vi "Forebrain.vi"() -> ()   [LabVIEW 2012]
doc: "This VI contrains the Forebrain within the Olin Robot Architecture. It must be run first to load the appropriate mission definition files. It contains a finite state machine built around a tabbed Operator interface that will guide an operator through the startup, run shutdown mission sequence. After running it, run the Midbrain and Hindbrain VIS."
panel:
  in  "Soft E-Stop":bool
  out "NXT String Received":string
  out "return count":u32
  out "error out":errorcluster
  in  "error in 2":errorcluster
  out "Desired \nVelocity":i16=5
  out "Local\nHeading":i16=90
  out "Ycurrent":dbl format="%#_3g"
  out "Xcurrent":dbl format="%#_3g"
  out "Ystart":dbl
  out "Xstart":dbl
  in  "error in":errorcluster
  out "Robot Live":bool
  in  "E-Stop":bool
  in  "Tab":T1(tab)
  out "MissionTime (Min)":dbl(knob) scale=0.0..10.0
  out "LidarDist":i16
  out "IR Index":i32
  out "BatteryLevel":dbl(slide) scale=6.0..9.0
  out "String Received":string
  out "Send String":string="$B^"
  in  "VISA resource name":refnum<visa-resource-name>="COM10"
  in  "Mode":i16 min=0 max=99 step=1
  in  "Desired Vel":i16(slide)=7 scale=0.0..14.0
  in  "Local Head":i16(slide)=7 scale=0.0..14.0
  out "StartMissionMap":picture
  out "MapDARCheck":picture
  in  "RunRobot":bool
  in  "Tug letter":string="G"
  out "Tug X":i32
  out "Tug Y":i32
  out "Tug H":i32
  out "BS Time Out?":bool
  out "Buoy locations":cluster{"regular expression":string, i32, i32}[](array[cluster])
  out "Valid ?":bool
  out "Battery\nVolts":i16
  out "Base Station data rec'd":string
  out "udp rate":bool
  out "CollisionWarning":bool
  out "DebugMapDAR":picture
  in  "MapDAR Control":T2={"NumberOfBeams"=180, "SensorRange"=500.0, "Noise (0.1 to 1)"=0.0} {"Noise (0.1 to 1)" min=0.0 max=1.0 step=0.1; "SensorRange" min=500.0 max=1500.0 step=100.0; "NumberOfBeams" min=36 max=360 step=2}
  out "MapDAR Data (r:pixel b:degrees)":cluster{"Range":dbl, "Bearing":dbl}[](array[cluster])
  in  "Stop DebugSENSE":bool
  out "MissionMap":picture
  out "Tug position":T3
  out "initialized MDF":T4(array[cluster])
  out "Way Point Index":i32
  out "InitialWaypoint":cluster{"X":i16, "Y":i16}
  in  "Pen Color":u32(colorbox)=15671808
  in  "Select Pen Attributes":T5={"Width"=1, "Style"=enum."Solid"}
  out "Draw??":bool
  in  "WhereAmI?FromBase":T6
  out "(xr,yr)":cluster{"X":dbl, "Y":dbl}
  in  "RobotPosition":T3 {"xrobot" min=0.0 max=1177.0 step=10.0; "yrobot" min=0.0 max=850.0 step=10.0; "heading" min=0.0 max=7.0 step=0.1}
  out "MDF_Original":T4(array[cluster])
  out "WhatAroundMeMap?":cluster{"T":dbl, "Range":dbl, "Bearing":dbl}[](array[cluster])
  out "WayPointAct":dbl[](array[numeric])
  out "SteerAngle":dbl
  out "MissionDefFile":picture
  out "MDF":T4(array[cluster])
  in  "Select Your Behavior":T7(ring)
  out "No. of Waypoints":i32
  in  "Exit Planning":bool
  in  "BoatSpeed for Leg":dbl(slide)=8.0 min=-9.0 max=9.0 step=1.0 scale=0.0..14.0
  out "BuildMDF":bool
  out "WayPoint Position":cluster{"X":i32, "Y":i32}
  in  "Upper Midbrain Active":bool
  out "Send String to NXT":string="$B^"
  in  "Behavior Command":T7(ring)
  out "CollisionLight":bool
  out "Where? Manual":T6
  out "ActManual":bool
  in  "Manual Heading":i16(knob) min=0 max=14 step=1
  out "MWhat?":bool
  out "Where? 2":bool
  out "How? 2":bool
  in  "ManualModeStop":bool
  out "ManualModeMapDAR":picture
  out "ManualMissionMap":picture
  out "Battery":dbl(slide) scale=0.0..8.0
  in  "Manual Vel":dbl(slide) min=0.0 max=14.0 step=1.0 scale=0.0..14.0
  out "MissionTime":dbl(knob) scale=0.0..10.0
  out "Heading":cluster{dbl, dbl}(knob)={0.0, 34.390870865624734} scale=180.0..-179.0 scale format="%#_3g"
  out "Speed":i16(knob) scale=-6.0..6.0
  out "Current Behavior":T7(ring)
  out "Robot Position":cluster{"X":dbl, "Y":dbl} {"X" format="%#_3g"; "Y" format="%#_3g"}
  out "Ready":bool
  in  "Pause":bool
  in  "Rerun MDF":bool
  out "CollisionLight 2":bool
  out "Act":bool
  out "Neo-C":bool
  out "How?":bool
  out "What?":bool
  out "A Heading":cluster{dbl, dbl}(knob)={0.0, 34.390870865624734} scale=180.0..-180.0
  out "A Speed":dbl(knob) scale=-9.0..9.0
  out "AutoBattery":dbl(slide) scale=0.0..8.0
  out "AutoModeLIDAR":picture
  out "AutoMissionMap":picture
  in  "RunAutoMode":bool
  out "MissionTimeAuto":dbl(knob) scale=0.0..60.0
  out "Where?":bool
  # "To run\nrobot,\nclick\narrow\nabove\n\nRun Robot button must be on"
  # "Operation Directions\n\n1)Click on Startup&\nShutdown tab.\n2) Click on Run \nArrow on menubar.\nRun Forebrain,\nvis from the project\nexplorer.\n3) Select a mssion \nmap file when asked.\n4) Check robot is \nfully operational on\nStartup tab.\n5) Debug with debug\ntabs as required.\n6) Select ManualMode\ntab and test drive \nrobot.\n7) Select PlanMission\ntab and set up \nmission.\n8) Go to AutoMode\ntab and run mission."
  # "Turns off drive\nmotors"
  # "Enter Olin Test  Pool"
  # "Xbee Com Port"
  # "xBee\"Send String\" (mode, desired velocity, local heading)"
  # "(Type in Tug Letter  L T G P  (look at boat cradle)"
  # "Should be on to\nrun"
  # "BoatG,X,Y,H,BoatT,X,Y,H,BoatP,X,Y.H,BoatL,X,Y,H,BuoyA,X,Y,BuoyB,X,Y,BuoyC,X,Y,BuoyD,X,Y,Time(hours,Min,Sec)"
  # "To stop  program \nturn off here"
  # "Use this tab\nto explore\nLIDAR\ndata and \noperation"
  # "Set\nNumberOfBeams\nSensorRange\nNoise\nto\nview\nsimulated\nsensor\ndata"
  # "Turn Debug Sim \nto leave this\ntab--->"
  # "This tab will auto\nreturn to Startup \nin 2 seconds"
  # "Clean up interface and make more useful for debugging behaviors"
  # "Build out interface and make more useful for debugging act"
  # "This tab will auto\nreturn to Startup \nin 2 seconds"
  # "Directions:\n1) Select Robot Behavior for each mission leg.\n2) Select Robot Speed for leg.\n3) Click on robots current location for first waypoint.\n4) Hold down button and drag to next\nwaypoint. Click on next leg waypoint.\n5) Hold mouse button down and drag to \nnext waypoint. \n6) Click on next waypoint. Repeat for full mission.\n7) MDF will store up to 20 waypoints."
  # "Remember to\nset boat\nleg speed !"
  # "Please Adjust Scroll Barrs in Tug Off Mode to Prevent  Extra Lines Being Drawn"
  # "\"Send String\" (mode, desired velocity, local heading)"
  # "Press to stop and return to StartUp"
  # "Open MidBrain\nArbiter to see\nBrain Waves"
  # "AutoMode\nAutomatically \nReturns to \nStartUp Mode"
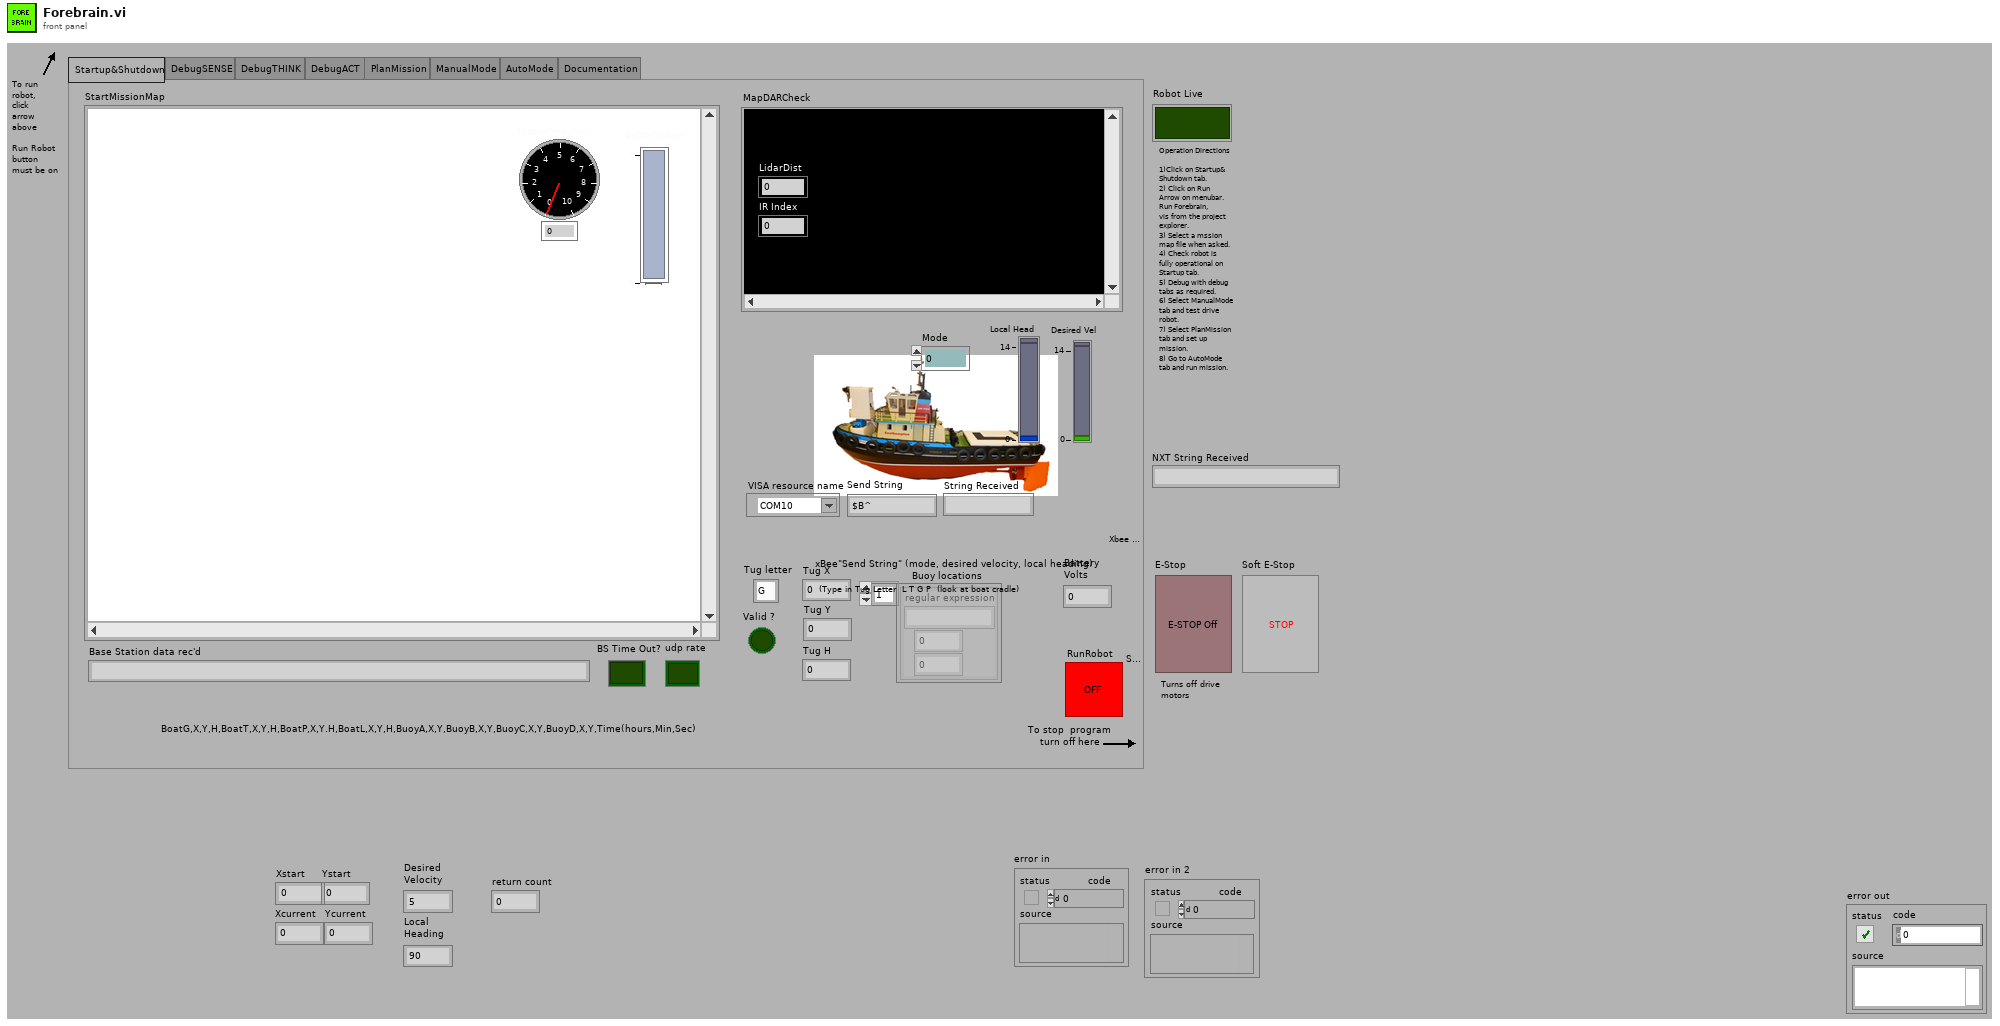
[diagram p1: front panel]
types:
  T1 = enum32{"Startup&Shutdown", "DebugSENSE", "DebugTHINK", "DebugACT", "PlanMission", "ManualMode", "AutoMode", "Documentation"}
  T2 = cluster{"NumberOfBeams":i32, "SensorRange":dbl, "Noise (0.1 to 1)":dbl}
  T3 = cluster{"xrobot":dbl, "yrobot":dbl, "heading":dbl}
  T4 = cluster{"Status":enum16{"Past", "Current", "Future"}, "x":dbl, "y":dbl, "z":dbl, "Vel":dbl, "Dwell Time":dbl, "BehCom":enum16{"Tug Off", "Manual Mode", "Goto WayPoint", "Back Up", "Circle", "Left Wall Follow", "Right Wall Follow", "Hunt"}, "Expand1":dbl, "Expand2":dbl, "Expand3":dbl}[]
  T5 = cluster{"Width":u16, "Style":enum32{"Solid", "Dash", "Dot", "DashDot", "DashDotDot"}}
  T6 = cluster{"T":dbl, "X":dbl, "Y":dbl, "Direction":dbl}
  T7 = enum16{"Tug Off", "Manual Mode", "Goto WayPoint", "Back Up", "Circle", "Left Wall Follow", "Right Wall Follow", "Hunt"}
  T8 = cluster{"VelCom":dbl, "BehCom":enum16{"OpenFieldTransit", "P-WallFollow", "S-WallFollow", "LaneFollow", "ManualMode"}}
  T9 = typedef "IMAQ Image.ctl" = refnum<image>
  T10 = typedef "imagedata.ctl" = cluster{"image type":i32, "image depth":i32, "image":u8[], "mask":u8[], "colors":u32[], "Rectangle":cluster{"left":i16, "top":i16, "right":i16, "bottom":i16}}
  T11 = cluster{"Status":enum16{"Past", "Current", "Future"}, "x":dbl, "y":dbl, "z":dbl, "Vel":dbl, "Dwell Time":dbl, "BehCom":enum16{"Tug Off", "Manual Mode", "Goto WayPoint", "Back Up", "Circle", "Left Wall Follow", "Right Wall Follow", "Hunt"}, "Expand1":dbl, "Expand2":dbl, "Expand3":dbl}
  T12 = typedef "LVMouseTypeDef.ctl" = cluster{"Mouse Position":cluster{"X":i32, "Y":i32}, "Mouse Modifiers":cluster{"Button Down":bool, "Shift Mod":bool, "Menu Mod":bool, "Option Mod":bool}}
  T13 = cluster{"regular expression":string, i32, i32, i32}
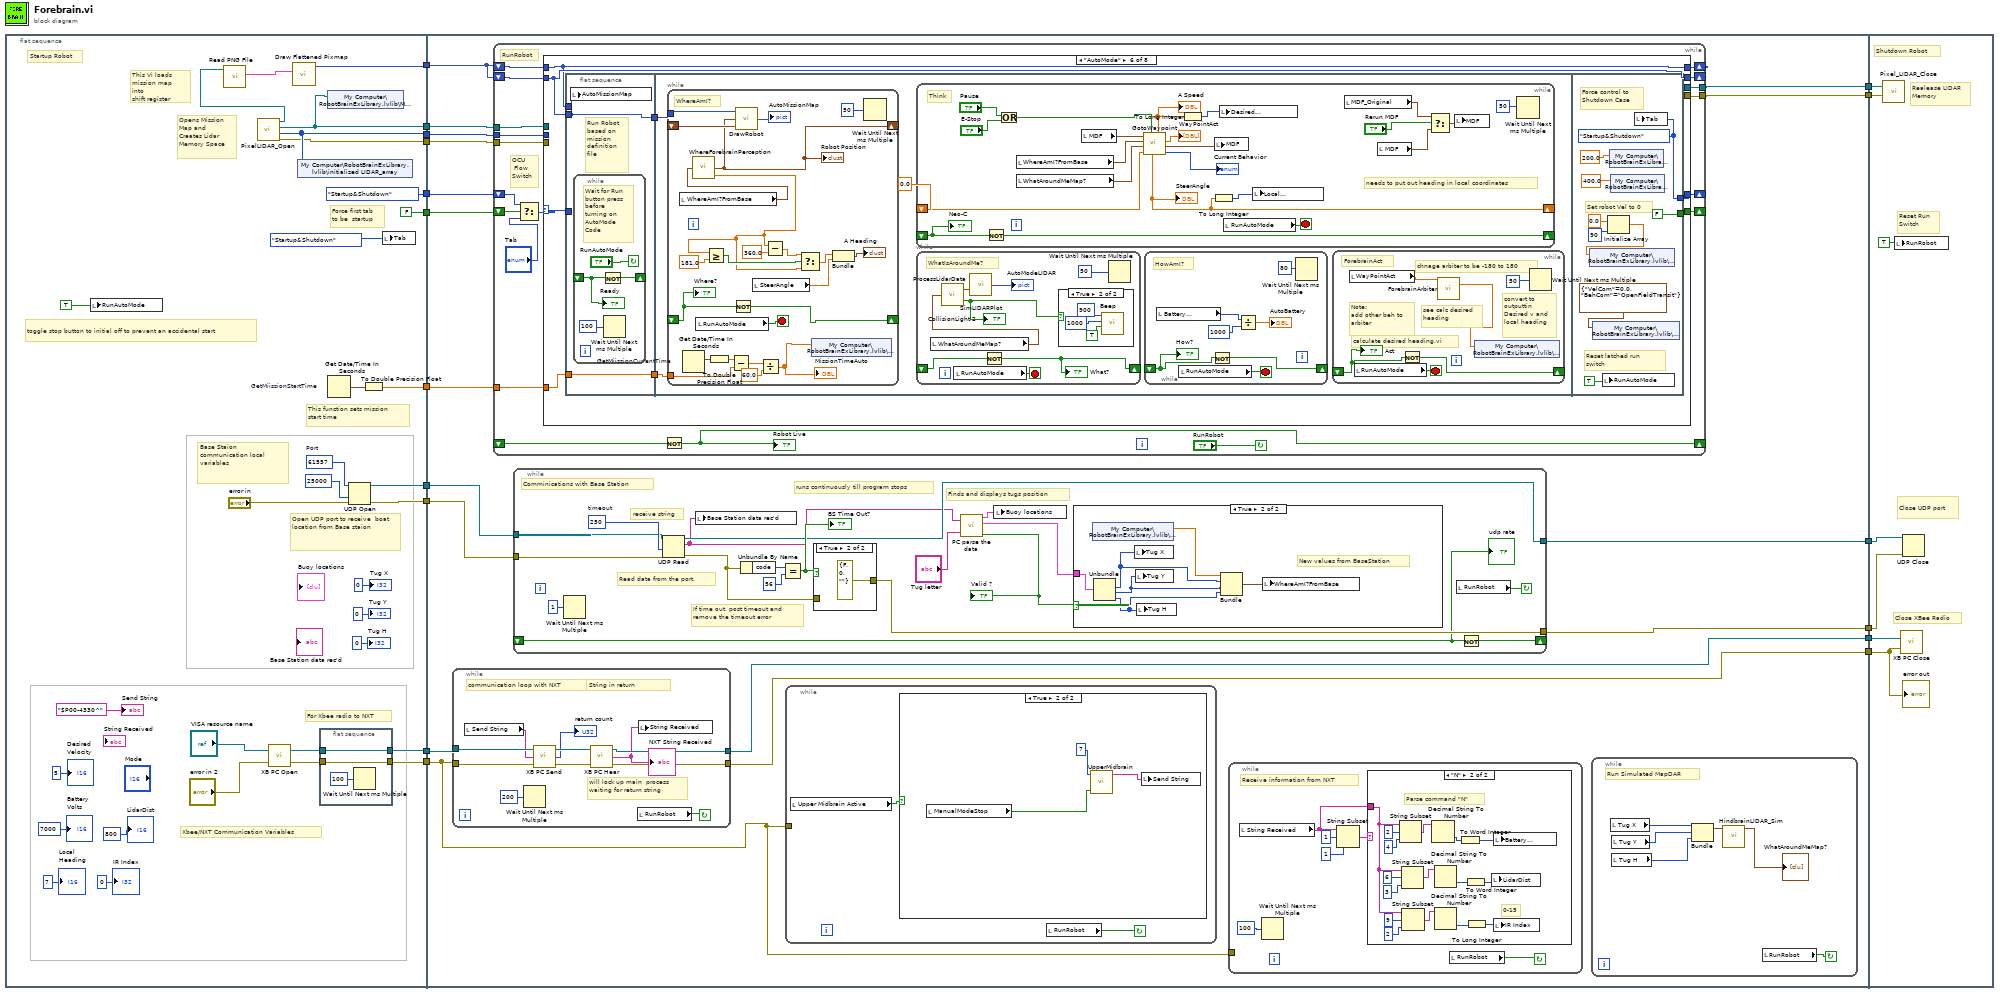
[diagram p0: block diagram]
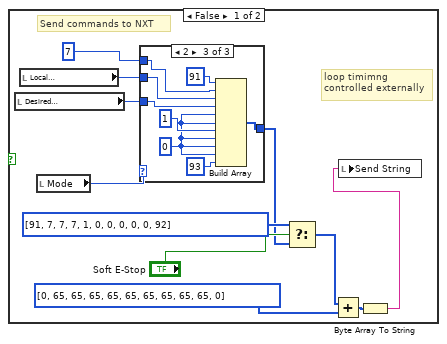
[diagram p3: hidden frame]
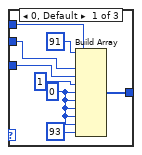
[diagram p4: hidden frame]
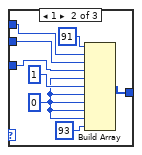
[diagram p5: hidden frame]
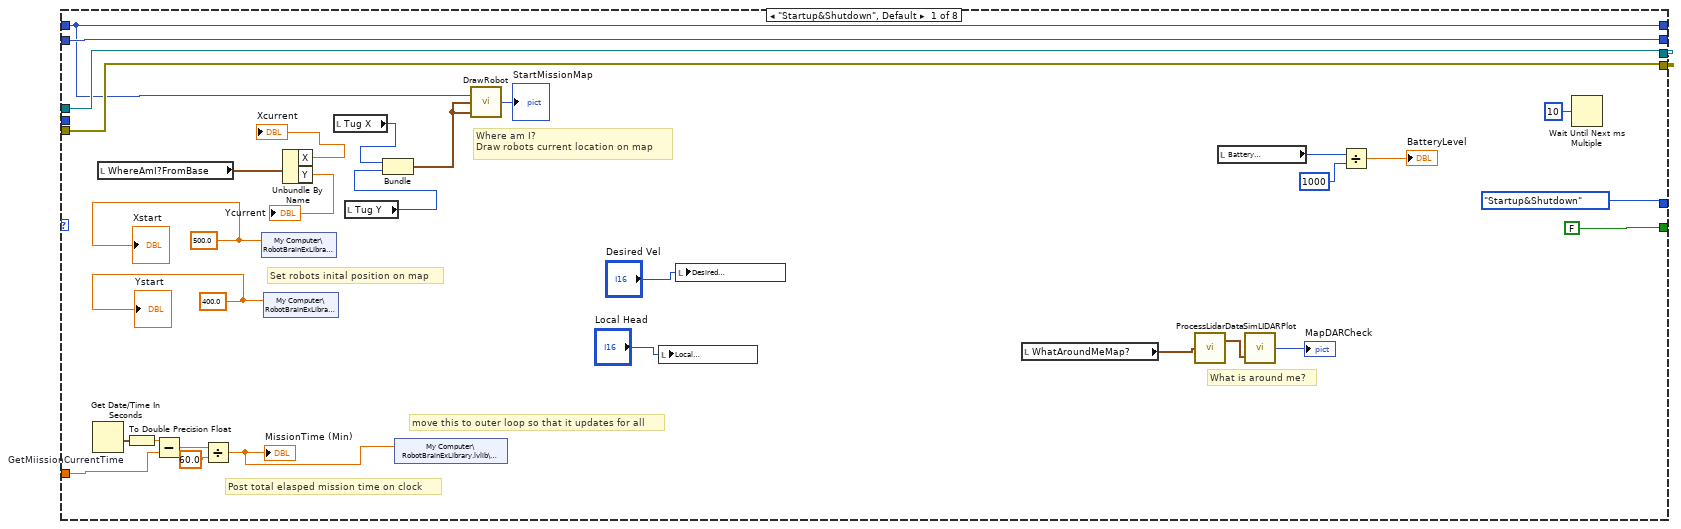
[diagram p8: hidden frame]
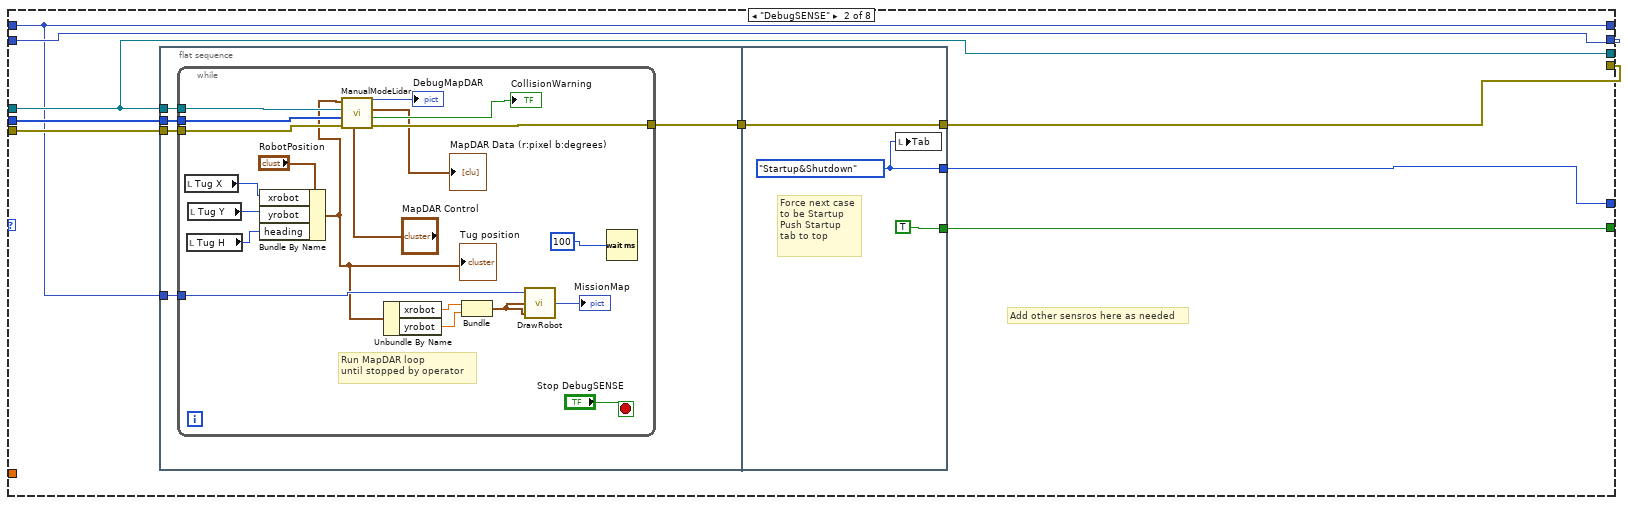
[diagram p9: hidden frame]
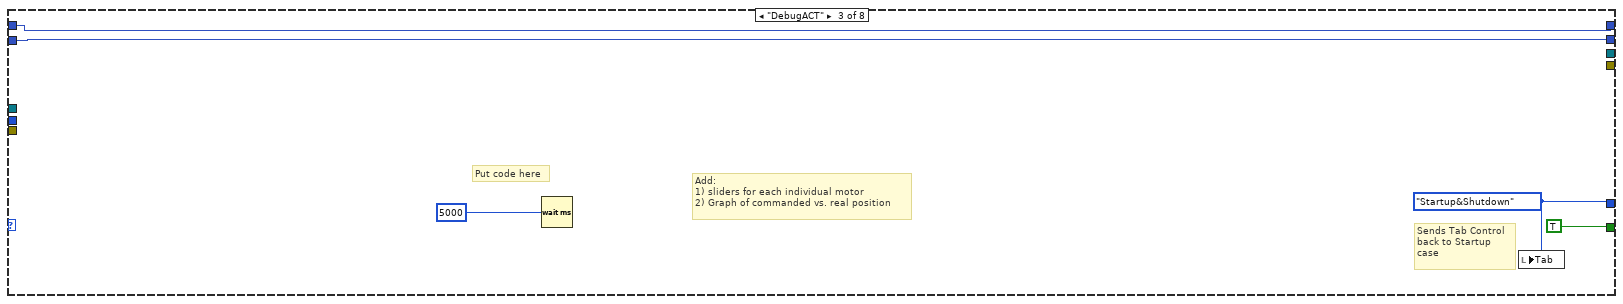
[diagram p10: hidden frame]
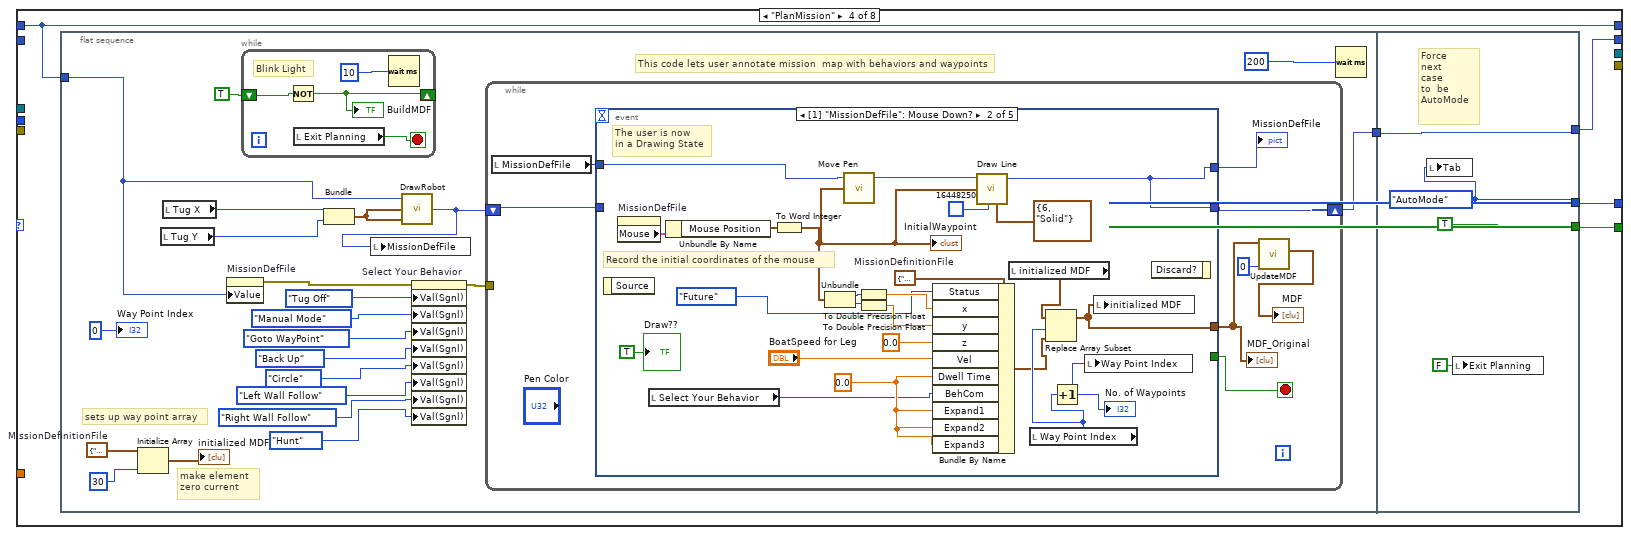
[diagram p11: hidden frame]
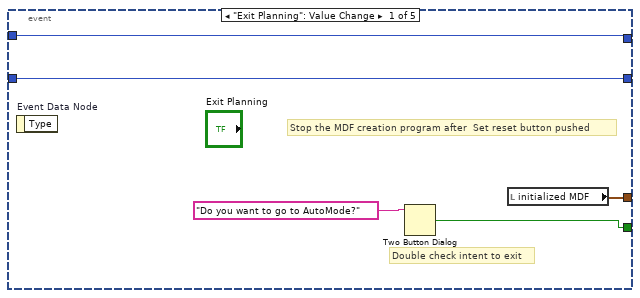
[diagram p12: hidden frame]
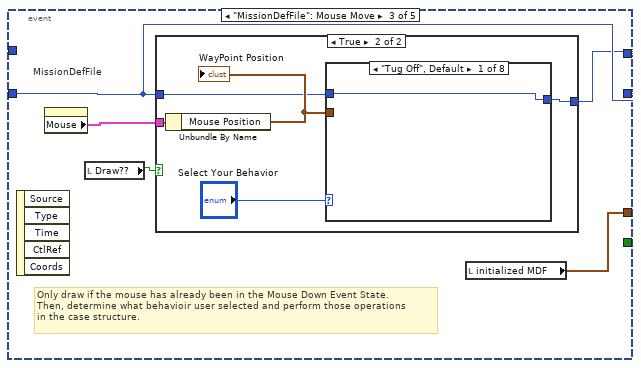
[diagram p13: hidden frame]
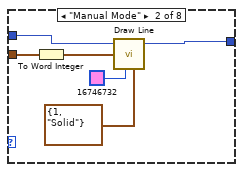
[diagram p15: hidden frame]
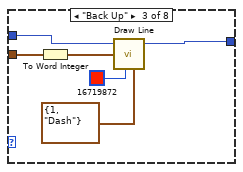
[diagram p16: hidden frame]
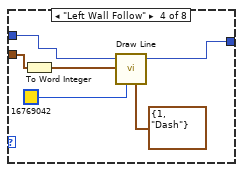
[diagram p17: hidden frame]
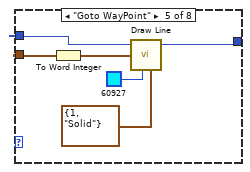
[diagram p18: hidden frame]
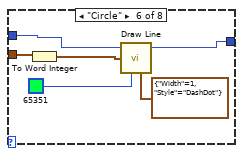
[diagram p19: hidden frame]
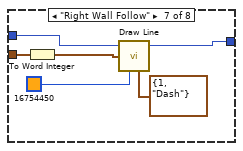
[diagram p20: hidden frame]
diagram:
  n1 = flat-sequence {
    tunnel: [w48] -> w17
    tunnel: [w47] -> w16
    tunnel: [w44] -> w15
    tunnel: [w46] -> w14
    tunnel: [w45] -> w13
    tunnel: [FALSE ("RunAutoMode")] -> w10
    tunnel: [T1."Startup&Shutdown" ("Tab")] -> w9
    tunnel: [w31] -> w8
    tunnel: [w30] -> w7
    tunnel: [w19] -> w6
    tunnel: [w18] -> w5
    tunnel: w17 -> [w69]
    tunnel: w16 -> [w68]
    tunnel: w15 -> [w67]
    tunnel: w14 -> [w66]
    tunnel: w13 -> [w65]
    tunnel: [w64] -> w12
    tunnel: [w63] -> w11
    tunnel: w10 -> [w62]
    tunnel: w9 -> [w61]
    tunnel: w8 -> [w56]
    tunnel: w7 -> [w55]
    tunnel: w6 -> [w60]
    tunnel: w5 -> [w57]
    tunnel: [w59] -> w4
    tunnel: [w58] -> w3
    tunnel: [w54] -> w2
    tunnel: [w53] -> w1
    tunnel: w12 -> [w616]
    tunnel: w11 -> [w615]
    tunnel: w4 -> [w614]
    tunnel: w3 -> [w613]
    tunnel: w2 -> [w612]
    tunnel: w1 -> [w611]
    frame #0 {
      w37 = u16 61557  # Port
      # "For Xbee radio to NXT"
      # "Xbee/NXT Communication Variables"
      # "Base Staion communication local variables"
      # "Open UDP port to receive  boat location from Base staion"
      # "Force first tab\nto be  startup"
      # "toggle stop button to initial off to prevent an accidental start"
      # "Opens Mission\nMap and\nCreates Lidar\nMemory Space"
      # "This function sets mission \nstart time"
      # "This Vi loads\nmission map into \nshift register"
      # "Startup Robot"
      n2 = local write "RunAutoMode"(TRUE ("RunAutoMode")) -> ()
      n3 = call "PixelLIDAR_Open.vi"() -> ("error out"=w45:errorcluster, "initialized LIDAR\narray"=w46:i32[], "MDF Image"=w44:T9, "MissionMap"=w39:path)  [unwired: 2 in]
      n4 = call <vilib>:"Read PNG File.vi"("path to PNG file"=w39) -> ("image data"=w38:T10)  [unwired: 8 in, 2 out]
      n5 = call "XB PC Open.vi"("error in (no error)"="error in 2", "VISA resource name"="VISA resource name") -> ("error out"=w22:errorcluster, "VISA resource name out"=w23:refnum<visa-resource-name>)
      n6 = call <vilib>:"Draw Flattened Pixmap.vi"("image data"=w38) -> ("new picture"=w47:picture)  [unwired: 8 in]
      n7 = shared-variable "My Computer\\RobotBrainExLibrary.lvlib\\initialized LIDAR_array"(w46) -> ()  [unwired: 1 in, 1 out]
      n8 = flat-sequence {
        tunnel: w23 -> [w50]
        tunnel: w22 -> [w51]
        tunnel: [w51] -> w18
        tunnel: [w50] -> w19
        frame #0 {
          n9 = Wait Until Next ms Multiple(millisecond multiple=u32 100) -> ()  [unwired: 1 out]
        }
      }
      n10 = shared-variable "My Computer\\RobotBrainExLibrary.lvlib\\MDF Image"(w44) -> ()  [unwired: 1 in, 1 out]
      n11 = Get Date/Time In Seconds "GetMiissionStartTime"() -> (seconds since 1Jan1904=w49:timestamp)
      n12 = UDP Open(8:"error in", 9:25000 ("timeout ms (25000)"), 11:w37) -> (port=w31:refnum<k16>, 0:w30:errorcluster)  [unwired: 2 in, 1 out]
      n13 = To Double Precision Float(number=w49) -> (double precision float=w48:dbl)
      n14 = local write "Tab"(T1."Startup&Shutdown" ("Tab")) -> ()
      "Tug X" <- 0 ("Tug X")
      "Tug Y" <- 0 ("Tug Y")
      "Tug H" <- 0 ("Tug H")
      "Battery\nVolts" <- i16 7000 ("Battery\nVolts")
      "LidarDist" <- i16 800 ("Dist")
      "IR Index" <- 0 ("IR Index")
      "Local\nHeading" <- i16 7 ("Local\nHeading")
      "Desired \nVelocity" <- i16 5 ("Desired \nVelocity")
      "Send String" <- "$P00-4330^"
    }
    frame #1 {
      n15 = while {
        tunnel: w60 -> [w148]
        tunnel: w57 -> [w147]
        tunnel: [w144] -> w58
        tunnel: [w143] -> w59
        stop <- w142 continue-if-true
        # "will lock up main  process\nwaiting for return string"
        # "communication loop with NXT"
        # "send a string to the NXT and receive a String in return"
        n16 = local read "Send String"() -> (w140:string)
        n17 = Wait Until Next ms Multiple(millisecond multiple=u32 200) -> ()  [unwired: 1 out]
        n18 = call "XB PC Send.vi"("error in (no error)"=w147, "String"=w140, "VISA resource name"=w148) -> ("error out"=w146:errorcluster, "return count"=→"return count":u32, "VISA resource name out"=w145:refnum<visa-resource-name>)
        n19 = call "XB PC Hear.vi"("VISA resource name"=w145, "error in (no error)"=w146) -> ("VISA resource name out"=w143:refnum<visa-resource-name>, "String Received"=w139:string, "error out"=w144:errorcluster)
        "NXT String Received" <- w139
        n20 = local read "RunRobot"() -> (w142:bool)
        n21 = local write "String Received"(w139) -> ()
      }
      n22 = while {
        shift-right: [w175] -> _
        shift-left: _ -> [w192]
        shift-right: [w191] -> _
        shift-left: w61 -> [w190]
        shift-right: [w187] -> _
        shift-left: w62 -> [w186]
        tunnel: w69 -> [w185]
        shift-right: [w183] -> _
        shift-left: w68 -> [w184]
        shift-right: [w181] -> _
        shift-left: w68 -> [w182]
        tunnel: w67 -> [w180]
        tunnel: w66 -> [w179]
        tunnel: w65 -> [w178]
        tunnel: [w177] -> w64
        tunnel: [w176] -> w63
        stop <- "RunRobot" continue-if-true
        # "RunRobot"
        # "OCU\n Flow\nSwitch"
        n23 = Select(t=w190, s=w186, f="Tab") -> (s? t:f=w188:T1)
        n24 = case shown="\"AutoMode\"" w188 {
          selector: w188 -> [_ _ _ _ _ w512 _ _]
          tunnel: [T1."Startup&Shutdown" ("Tab") w228 w263 w270 w437 w513 T1."Startup&Shutdown" ("Tab") w609] -> w191
          tunnel: [FALSE ("s") w227 TRUE ("s") w269 w438 w511 FALSE ("s") TRUE ("s")] -> w187
          tunnel: w185 -> [w217 _ _ _ w435 w509 _ _]
          tunnel: w184 -> [w210 w224 w262 w266 w433 w506 w602 w607]
          tunnel: [w210 w224 w262 w266 w433 w506 w602 w607] -> w183
          tunnel: w182 -> [w216 w225 w261 _ w434 w508 w601 w606]
          tunnel: [w216 w225 w261 w267 w434 w508 w601 w606] -> w181
          tunnel: w180 -> [w215 w226 _ _ _ _ _ _]
          tunnel: w179 -> [_ w232 _ _ _ _ _ _]
          tunnel: w178 -> [w214 w231 _ _ _ _ _ _]
          tunnel: [w215 w226 _ _ _ _ _ _] -> w177
          tunnel: [w214 w230 _ _ _ _ _ _] -> w176
          frame "Startup&Shutdown", Default {
            w205 = 400.0 ("Ystart")
            w206 = 500.0 ("Xstart")
            # "move this to outer loop so that it updates for all"
            # "Where am I?\nDraw robots current location on map"
            # "Post total elasped mission time on clock"
            # "What is around me?"
            # "Set robots inital position on map"
            n25 = Get Date/Time In Seconds "GetMiissionCurrentTime"() -> (seconds since 1Jan1904=w221:timestamp)
            n26 = local read "WhereAmI?FromBase"() -> (w194:T6)
            n27 = To Double Precision Float(number=w221) -> (double precision float=w220:dbl)
            n28 = Subtract(x=w220, y=w217) -> (x-y=w219:dbl)
            n29 = Divide(x=w219, y=60.0) -> (x/y=w213:dbl)
            "MissionTime (Min)" <- w213
            n30 = shared-variable "My Computer\\RobotBrainExLibrary.lvlib\\Xstart"(w206) -> ()  [unwired: 1 in, 1 out]
            n31 = shared-variable "My Computer\\RobotBrainExLibrary.lvlib\\Ystart"(w205) -> ()  [unwired: 1 in, 1 out]
            n32 = Unbundle By Name(w194) -> ("X"=→"Xcurrent":dbl, "Y"=→"Ycurrent":dbl)
            n33 = local read "Tug X"() -> (w204:i32)
            n34 = local read "Tug Y"() -> (w203:i32)
            n35 = Bundle("Tug X"=w204, "Tug Y"=w203) -> (w209:cluster{"Tug X":i32, "Tug Y":i32})  [unwired: 1 in]
            n36 = shared-variable "My Computer\\RobotBrainExLibrary.lvlib\\MissionTime"(w213) -> ()  [unwired: 1 in, 1 out]
            n37 = call "DrawRobot.vi"("(xr,yr) old"=w209, "(xr,yr) new"=w209, "2D Picture"=w210) -> ("new picture"=→"StartMissionMap":picture)
            n38 = local write "Local\nHeading"("Local Head") -> ()
            n39 = local write "Desired \nVelocity"("Desired Vel") -> ()
            n40 = local read "WhatAroundMeMap?"() -> (w195:cluster{"T":dbl, "Range":dbl, "Bearing":dbl}[])
            n41 = call "ProcessLidarData.vi"("WhatAroundMe?MM"=w195) -> ("data array [mag, phase (deg)]"=w211:cluster{"magnitude":dbl, "phase":dbl}[])  [unwired: 1 out]
            n42 = local read "Battery\nVolts"() -> (w200:i16)
            n43 = call "SimLIDARPlot.vi"("data array [mag, phase (deg)]"=w211) -> ("SONAR"=→"MapDARCheck":picture)  [unwired: 1 in]
            n44 = Divide(x=w200, y=i16 1000) -> (x/y=→"BatteryLevel":dbl)
            n45 = Wait Until Next ms Multiple(millisecond multiple=u32 10) -> ()  [unwired: 1 out]
            "Xstart" <- w206
            "Ystart" <- w205
          }
          frame "DebugSENSE" {
            # "Add other sensros here as needed"
            n46 = flat-sequence {
              tunnel: w232 -> [w237]
              tunnel: w231 -> [w236]
              tunnel: w226 -> [w235]
              tunnel: [w234] -> w229
              tunnel: w224 -> [w233]
              tunnel: [w260] -> w230
              tunnel: w229 -> [w260]
              tunnel: [w259] -> w228
              tunnel: [TRUE ("s")] -> w227
              frame #0 {
                n47 = while {
                  tunnel: w237 -> [w257]
                  tunnel: w236 -> [w256]
                  tunnel: w235 -> [w255]
                  tunnel: [w254] -> w234
                  tunnel: w233 -> [w248]
                  stop <- "Stop DebugSENSE" stop-if-true
                  # "Run MapDAR loop\nuntil stopped by operator"
                  n48 = local read "Tug X"() -> (w242:i32)
                  n49 = local read "Tug H"() -> (w243:i32)
                  n50 = local read "Tug Y"() -> (w241:i32)
                  n51 = Bundle By Name(cluster="RobotPosition", "xrobot"=w242, "yrobot"=w241, "heading"=w243) -> (w239:T3)
                  "Tug position" <- w239
                  n52 = call "ManualModeLidar.vi"("LIDARControl"="MapDAR Control", "error in"=w256, "initialized \nsonar ray\narray"=w257, "MDF Image"=w255, "SubPosition"=w239) -> ("error out"=w254:errorcluster, "Collision\nWarning"=→"CollisionWarning":bool, "LIDAR Data (r:pixel b:degrees)"=→"MapDAR Data (r:pixel b:degrees)":cluster{"Range":dbl, "Bearing":dbl}[], "LIDAR"=→"DebugMapDAR":picture)  [unwired: 1 in]
                  n53 = Unbundle By Name(w239) -> ("xrobot"=w246:dbl, "yrobot"=w245:dbl)
                  n54 = Bundle("xrobot"=w246, "yrobot"=w245) -> (w238:cluster{"xrobot":dbl, "yrobot":dbl})  [unwired: 1 in]
                  n55 = call "DrawRobot.vi"("(xr,yr) old"=w238, "(xr,yr) new"=w238, "2D Picture"=w248) -> ("new picture"=→"MissionMap":picture)
                  n56 = Wait (ms)(milliseconds to wait=u32 100) -> ()  [unwired: 1 out]
                }
              }
              frame #1 {
                w259 = T1."Startup&Shutdown" ("Tab")
                # "Force next case\nto be Startup\nPush Startup\ntab to top"
                n57 = local write "Tab"(w259) -> ()
              }
            }
          }
          frame "DebugACT" {
            w263 = T1."Startup&Shutdown" ("Tab")
            # "Add:\n1) sliders for each individual motor\n2) Graph of commanded vs. real position"
            # "Put code here"
            # "Sends Tab Control\nback to Startup\ncase"
            n58 = Wait (ms)(milliseconds to wait=u32 5000) -> ()  [unwired: 1 out]
            n59 = local write "Tab"(w263) -> ()
          }
          frame "PlanMission" {
            n60 = flat-sequence {
              tunnel: [w291] -> w268
              tunnel: w266 -> [w284]
              tunnel: [w431] -> w270
              tunnel: [TRUE ("s")] -> w269
              tunnel: w268 -> [w430]
              tunnel: [w430] -> w267
              frame #0 {
                w282 = T11 {"Status"=enum."Future", "x"=0.0, "y"=0.0, "z"=0.0, "Vel"=0.0, "Dwell Time"=0.0, "BehCom"=enum."Tug Off", "Expand1"=0.0, "Expand2"=0.0, "Expand3"=0.0}  # MissionDefinitionFile
                # "make element \nzero current"
                # "sets up way point array"
                # "This code lets user annotate mission  map with behaviors and waypoints"
                n61 = Initialize Array ("Initialize WaypointArray")(w282, 30 ("dimension size")) -> (→"initialized MDF":T4)
                n62 = local read "Tug Y"() -> (w279:i32)
                n63 = local read "Tug X"() -> (w280:i32)
                n64 = property on="MissionDefFile" class="Pict"("Value"=w284) -> (error out=w289:errorcluster)  [unwired: 2 in, 1 out]
                n65 = while {
                  shift-right: [w295] -> _
                  shift-left: TRUE -> [w296]
                  stop <- w294 stop-if-true
                  # "Blink Light"
                  n66 = Not(x=w296) -> (.not. x?=w295:bool)
                  "BuildMDF" <- w295
                  n67 = local read "Exit Planning"() -> (w294:bool)
                  n68 = Wait (ms)(milliseconds to wait=u32 10) -> ()  [unwired: 1 out]
                }
                n69 = Bundle("Tug X"=w280, "Tug Y"=w279) -> (w285:cluster{"Tug X":i32, "Tug Y":i32})  [unwired: 1 in]
                n70 = call "DrawRobot.vi"("(xr,yr) old"=w285, "(xr,yr) new"=w285, "2D Picture"=w284) -> ("new picture"=w283:picture)
                n71 = local write "MissionDefFile"(w283) -> ()
                n72 = property on="Select Your Behavior" class="Enum (strict)"(error in=w289, "Val(Sgnl)"=T7."Tug Off" ("Value (Signaling)"), "Val(Sgnl)"=T7."Manual Mode" ("Value (Signaling)"), "Val(Sgnl)"=T7."Goto WayPoint" ("Value (Signaling)"), "Val(Sgnl)"=T7."Back Up" ("Value (Signaling)"), "Val(Sgnl)"=T7."Circle" ("Value (Signaling)"), "Val(Sgnl)"=T7."Left Wall Follow" ("Value (Signaling)"), "Val(Sgnl)"=T7."Right Wall Follow" ("Value (Signaling)"), "Val(Sgnl)"=T7."Hunt" ("Value (Signaling)")) -> (error out=w290:errorcluster)  [unwired: 1 in, 1 out]
                n73 = while {
                  shift-right: [w303] -> w291
                  shift-left: w283 -> [w304]
                  tunnel: w290 -> [_]
                  stop <- w302 stop-if-true
                  n74 = local read "MissionDefFile"() -> (w301:picture)
                  n75 = event shown="[1] \"MissionDefFile\": Mouse Down?" {
                    selector: _ -> [_ _ _ _ _]
                    dyn-events: _ -> [_ _ _ _ _]
                    timeout: _ -> [_ _ _ _ _]
                    tunnel: [w307 w315 w335 w388 w426] -> w303
                    tunnel: w304 -> [w307 _ w335 w388 _]
                    tunnel: [w308 _ _ _ _] -> w302
                    tunnel: [w306 w330 w336 w390 w427] -> w298
                    tunnel: w301 -> [w305 w316 _ w389 w426]
                    tunnel: [w305 w315 w334 w389 w426] -> w300
                    event "Exit Planning": Value Change {
                      # "Double check intent to exit"
                      # "Stop the MDF creation program after  Set reset button pushed"
                      n76 = event-data "Event Data Node"() -> ()  [unwired: 1 in, 1 out]
                      n77 = Two Button Dialog(message="Do you want to go to AutoMode?") -> (T button?=w308:bool)  [unwired: 2 in]
                      n78 = local read "initialized MDF"() -> (w306:T4)
                    }
                    event "MissionDefFile": Mouse Down? {
                      w314 = T11 {"Status"=enum."Future", "x"=0.0, "y"=0.0, "z"=0.0, "Vel"=0.0, "Dwell Time"=0.0, "BehCom"=enum."Tug Off", "Expand1"=0.0, "Expand2"=0.0, "Expand3"=0.0}  # MissionDefinitionFile
                      w324 = 0.0 ("Dwell Time")
                      # "Record the initial coordinates of the mouse"
                      # "The user is now\nin a Drawing State"
                      n79 = event-data() -> ()  [unwired: 1 in, 1 out]
                      n80 = property on="MissionDefFile" class="Pict"() -> ("Mouse"=w333:T12)  [unwired: 2 in, 2 out]
                      n81 = local read "Select Your Behavior"() -> (w311:T7)
                      n82 = Unbundle By Name(w333) -> ("Mouse Position"=w331:cluster{"X":i32, "Y":i32})
                      n83 = To Word Integer(number=w331) -> (16bit integer=w319:cluster{"X":i16, "Y":i16})
                      "InitialWaypoint" <- w319
                      n84 = Unbundle(w319) -> ("X"=w328:i16, "Y"=w327:i16)
                      n85 = call <vilib>:"Move Pen.vi"("new position"=w319, "picture"=w316) -> ("new picture"=w320:picture)  [unwired: 3 in]
                      n86 = To Double Precision Float(number=w328) -> (double precision float=w326:dbl)
                      n87 = To Double Precision Float(number=w327) -> (double precision float=w325:dbl)
                      n88 = Bundle By Name(cluster=w314, "Status"=enum16{"Past", "Current", "Future"}."Future", "x"=w326, "y"=w325, "z"=0.0, "Vel"="BoatSpeed for Leg", "Dwell Time"=w324, "BehCom"=w311, "Expand1"=w324, "Expand2"=w324, "Expand3"=w324) -> (w310:T11)
                      n89 = call <vilib>:"Draw Line.vi"("picture"=w320, "end point"=w319, "color(black)"=u32 16448250, "pen"=T5 {"Width"=6, "Style"=enum."Solid"}) -> ("new picture"=w315:picture)  [unwired: 5 in]
                      n90 = local read "initialized MDF"() -> (w329:T4)
                      n91 = local read "Way Point Index"() -> (w312:i32)
                      n92 = Replace Array Subset(array=w329, new element=w310, index=w312) -> (w330:T4)
                      n93 = Increment(x=w312) -> (x+1=w332:i32)
                      "No. of Waypoints" <- w332
                      n94 = local write "Way Point Index"(w332) -> ()
                      n95 = local write "initialized MDF"(w330) -> ()
                      n96 = event-data() -> ()  [unwired: 2 in, 1 out]
                      "Draw??" <- TRUE ("Draw??")
                    }
                    event "MissionDefFile": Mouse Move {
                      # "Only draw if the mouse has already been in the Mouse Down Event State.\nThen, determine what behavioir user selected and perform those operations\nin the case structure."
                      n97 = event-data() -> ()  [unwired: 1 in, 5 out]
                      n98 = property on="MissionDefFile" class="Pict"() -> ("Mouse"=w338:T12)  [unwired: 2 in, 2 out]
                      n99 = local read "Draw??"() -> (w337:bool)
                      n100 = case shown="True" w337 {
                        tunnel: w338 -> [_ w344]
                        tunnel: w335 -> [w339 w340]
                        tunnel: [w339 w341] -> w334
                        frame False {
                        }
                        frame True {
                          n101 = Unbundle By Name(w344) -> ("Mouse Position"=w342:cluster{"X":i32, "Y":i32})
                          "WayPoint Position" <- w342
                          n102 = case shown="\"Tug Off\", Default" "Select Your Behavior" {
                            tunnel: w342 -> [_ w350 w356 w359 w365 w370 w376 w382]
                            tunnel: [w345 w351 w357 w361 w364 w371 w377 w383] -> w341
                            tunnel: w340 -> [w345 w349 w353 w362 w366 w372 w378 w384]
                            frame "Tug Off", Default {
                            }
                            frame "Manual Mode" {
                              n103 = To Word Integer(number=w350) -> (16bit integer=w346:cluster{"X":i16, "Y":i16})
                              n104 = call <vilib>:"Draw Line.vi"("picture"=w349, "end point"=w346, "color(black)"=u32 16746732, "pen"=T5 {"Width"=1, "Style"=enum."Solid"}) -> ("new picture"=w351:picture)  [unwired: 5 in]
                            }
                            frame "Back Up" {
                              n105 = To Word Integer(number=w356) -> (16bit integer=w352:cluster{"X":i16, "Y":i16})
                              n106 = call <vilib>:"Draw Line.vi"("picture"=w353, "end point"=w352, "color(black)"=u32 16719872, "pen"=T5 {"Width"=1, "Style"=enum."Dash"}) -> ("new picture"=w357:picture)  [unwired: 5 in]
                            }
                            frame "Left Wall Follow" {
                              n107 = To Word Integer(number=w359) -> (16bit integer=w360:cluster{"X":i16, "Y":i16})
                              n108 = call <vilib>:"Draw Line.vi"("picture"=w362, "end point"=w360, "color(black)"=u32 16769042, "pen"=T5 {"Width"=1, "Style"=enum."Dash"}) -> ("new picture"=w361:picture)  [unwired: 5 in]
                            }
                            frame "Goto WayPoint" {
                              n109 = To Word Integer(number=w365) -> (16bit integer=w367:cluster{"X":i16, "Y":i16})
                              n110 = call <vilib>:"Draw Line.vi"("picture"=w366, "end point"=w367, "color(black)"=u32 60927, "pen"=T5 {"Width"=1, "Style"=enum."Solid"}) -> ("new picture"=w364:picture)  [unwired: 5 in]
                            }
                            frame "Circle" {
                              n111 = To Word Integer(number=w370) -> (16bit integer=w375:cluster{"X":i16, "Y":i16})
                              n112 = call <vilib>:"Draw Line.vi"("picture"=w372, "end point"=w375, "color(black)"=u32 65351, "pen"=T5 {"Width"=1, "Style"=enum."DashDot"}) -> ("new picture"=w371:picture)  [unwired: 5 in]
                            }
                            frame "Right Wall Follow" {
                              n113 = To Word Integer(number=w376) -> (16bit integer=w381:cluster{"X":i16, "Y":i16})
                              n114 = call <vilib>:"Draw Line.vi"("picture"=w378, "end point"=w381, "color(black)"=u32 16754450, "pen"=T5 {"Width"=1, "Style"=enum."Dash"}) -> ("new picture"=w377:picture)  [unwired: 5 in]
                            }
                            frame "Hunt" {
                              n115 = To Word Integer(number=w382) -> (16bit integer=w385:cluster{"X":i16, "Y":i16})
                              n116 = call <vilib>:"Draw Line.vi"("picture"=w384, "end point"=w385, "color(black)"=u32 16720896, "pen"=T5 {"Width"=1, "Style"=enum."DashDotDot"}) -> ("new picture"=w383:picture)  [unwired: 5 in]
                            }
                          }
                        }
                      }
                      n117 = local read "initialized MDF"() -> (w336:T4)
                    }
                    event "Select Your Behavior": Value Change {
                      # "When the user selects a new operation, we disable certain controls that aren't relevant to\nthe operation that the user is performing."
                      n118 = event-data() -> ("NewVal"=w393:T7)  [unwired: 1 in]
                      n119 = property on="Select Pen Attributes" class="Clust (strict)"() -> ("Controls[]"=w392:refnum<vi>[])  [unwired: 2 in, 2 out]
                      n120 = case shown="\"Manual Mode\"" w393 {
                        tunnel: w392 -> [w397 w398 w402 w406 w410 w414 w418 w422]
                        tunnel: "Select Pen Attributes" -> [_ _ _ _ _ _ _ _]
                        frame "Manual Mode" {
                          # "All attributes are valid for this\noperation."
                          n121 = Index Array "Index Array"(array=w397, index=1) -> (element=w395:refnum<vi>)
                          n122 = property on="Property Node" class="Ctl"(reference=w395, "Disabled"=u8 0) -> ()  [unwired: 1 in, 2 out]
                        }
                        frame "Back Up" {
                          # "All attributes are valid for this\noperation."
                          n123 = Index Array(array=w398, index=1) -> (element=w400:refnum<vi>)
                          n124 = property class="Ctl"(reference=w400, "Disabled"=u8 0) -> ()  [unwired: 1 in, 2 out]
                        }
                        frame "Tug Off" {
                          # "All attributes are valid for this\noperation."
                          n125 = Index Array "Index Array"(array=w402, index=1) -> (element=w404:refnum<vi>)
                          n126 = property on="Property Node" class="Ctl"(reference=w404, "Disabled"=u8 0) -> ()  [unwired: 1 in, 2 out]
                        }
                        frame "Left Wall Follow" {
                          # "All attributes are valid for this\noperation."
                          n127 = Index Array "Index Array"(array=w406, index=1) -> (element=w408:refnum<vi>)
                          n128 = property on="Property Node" class="Ctl"(reference=w408, "Disabled"=u8 0) -> ()  [unwired: 1 in, 2 out]
                        }
                        frame "Goto WayPoint" {
                          # "All attributes are valid for this\noperation."
                          n129 = Index Array "Index Array"(array=w410, index=1) -> (element=w412:refnum<vi>)
                          n130 = property on="Property Node" class="Ctl"(reference=w412, "Disabled"=u8 0) -> ()  [unwired: 1 in, 2 out]
                        }
                        frame "Circle" {
                          # "All attributes are valid for this\noperation."
                          n131 = Index Array "Index Array"(array=w414, index=1) -> (element=w416:refnum<vi>)
                          n132 = property on="Property Node" class="Ctl"(reference=w416, "Disabled"=u8 0) -> ()  [unwired: 1 in, 2 out]
                        }
                        frame "Right Wall Follow" {
                          # "All attributes are valid for this\noperation."
                          n133 = Index Array "Index Array"(array=w418, index=1) -> (element=w420:refnum<vi>)
                          n134 = property on="Property Node" class="Ctl"(reference=w420, "Disabled"=u8 0) -> ()  [unwired: 1 in, 2 out]
                        }
                        frame "Hunt" {
                          # "All attributes are valid for this\noperation."
                          n135 = Index Array "Index Array"(array=w422, index=1) -> (element=w424:refnum<vi>)
                          n136 = property on="Property Node" class="Ctl"(reference=w424, "Disabled"=u8 0) -> ()  [unwired: 1 in, 2 out]
                        }
                      }
                      n137 = local read "initialized MDF"() -> (w390:T4)
                    }
                    event "MissionDefFile": Mouse Up {
                      # "When the user is finished drawing, we complete the operation."
                      # "Finished Drawing"
                      n138 = event-data() -> ()  [unwired: 1 in, 3 out]
                      n139 = local write "Draw??"(FALSE ("Draw??")) -> ()
                      n140 = local read "initialized MDF"() -> (w427:T4)
                    }
                  }
                  "MissionDefFile" <- w300
                  "MDF_Original" <- w298
                  n141 = call "UpdateMDF.vi"("Index"=0, "MDF_In"=w298) -> ("MDF_Out"=→"MDF":T4)  [unwired: 9 in]
                }
                n142 = Wait (ms)(milliseconds to wait=u32 200) -> ()  [unwired: 1 out]
                "Way Point Index" <- 0 ("Boundary Point Index")
              }
              frame #1 {
                w431 = T1."AutoMode" ("Tab")
                # "Force \nnext \ncase\nto  be\nAutoMode"
                n143 = local write "Tab"(w431) -> ()
                n144 = local write "Exit Planning"(FALSE ("Exit Planning")) -> ()
              }
            }
          }
          frame "ManualMode" {
            # "Removing map shift register\nfixed memory leak?"
            # "Manual Steering by dashboard heading steering wheel\nand by speed slider"
            # "This mode lets \noperator directly\ndrive robot via\nthe ManualMode\ntabbed interface"
            n145 = while {
              shift-right: [w461] -> _
              shift-left: _ -> [w460]
              tunnel: w435 -> [w453]
              shift-right: [w450] -> _
              shift-left: _ -> [w449]
              tunnel: w433 -> [w447]
              stop <- w459 stop-if-true
              # "WhereAmI?"
              n146 = Get Date/Time In Seconds "GetMiissionCurrentTime"() -> (seconds since 1Jan1904=w454:timestamp)
              n147 = call "WhereForebrainPerception.vi"("Where? Midbrain"="WhereAmI?FromBase") -> ("Where? Forebrain"=→"Where? Manual":T6, "(xr,yr)"=w450:cluster{"X":dbl, "Y":dbl}, "Direction"=w439:dbl)  [unwired: 3 in, 1 out]
              "(xr,yr)" <- w450
              n148 = local read "ManualModeStop"() -> (w459:bool)
              n149 = To Double Precision Float(number=w454) -> (double precision float=w455:dbl)
              n150 = Greater Or Equal?(x=w439, y=181.0) -> (x >= y?=w444:bool)
              n151 = local read "Manual Heading"() -> (w451:i16)
              n152 = Subtract(x=w455, y=w453) -> (x-y=w456:dbl)
              n153 = Not(x=w460) -> (.not. x?=w461:bool)
              n154 = call "DrawRobot.vi"("(xr,yr) old"=w449, "(xr,yr) new"=w450, "2D Picture"=w447) -> ("new picture"=→"ManualMissionMap":picture)
              n155 = Divide(x=w456, y=60.0) -> (x/y=w458:dbl)
              "MissionTime" <- w458
              n156 = Subtract(x=w439, y=360.0) -> (x-y=w442:dbl)
              n157 = shared-variable "My Computer\\RobotBrainExLibrary.lvlib\\MissionTime"(w458) -> ()  [unwired: 1 in, 1 out]
              n158 = Select(t=w442, s=w444, f=w439) -> (s? t:f=w441:dbl)
              n159 = Bundle("Direction"=w441, "Manual Heading"=w451) -> (→"Heading":cluster{"Direction":dbl, "Manual Heading":i16})  [unwired: 1 in]
              n160 = Wait Until Next ms Multiple(millisecond multiple=u32 100 ("milliseconds to wait")) -> ()  [unwired: 1 out]
              "Where? 2" <- w460
            }
            n161 = while {
              shift-right: [w468] -> _
              shift-left: _ -> [w469]
              stop <- "ManualModeStop" stop-if-true
              # "WhatIsAroundMe?"
              n162 = local read "WhatAroundMeMap?"() -> (w463:cluster{"T":dbl, "Range":dbl, "Bearing":dbl}[])
              n163 = call "ProcessLidarData.vi"("WhatAroundMe?MM"=w463) -> ("Collision"=w464:bool, "data array [mag, phase (deg)]"=w465:cluster{"magnitude":dbl, "phase":dbl}[])
              "CollisionLight" <- w464
              n164 = Not(x=w469) -> (.not. x?=w468:bool)
              "MWhat?" <- w468
              n165 = call "SimLIDARPlot.vi"("data array [mag, phase (deg)]"=w465) -> ("SONAR"=→"ManualModeMapDAR":picture)  [unwired: 1 in]
              n166 = case shown="True" w464 {
                frame False {
                  # "No \nBeep"
                }
                frame True {
                  n167 = call <vilib>:"Beep.vi"("use system alert? (T)"=TRUE, "duration (msec)"=u32 1000, "frequency (Hz)"=u32 900) -> ()  [unwired: 9 in]
                }
              }
              n168 = Wait Until Next ms Multiple(millisecond multiple=u32 100 ("milliseconds to wait")) -> ()  [unwired: 1 out]
            }
            n169 = while {
              shift-right: [w493] -> _
              shift-left: _ -> [w492]
              stop <- w491 stop-if-true
              # "HowAmI?"
              n170 = local read "Battery\nVolts"() -> (w490:i16)
              n171 = local read "ManualModeStop"() -> (w491:bool)
              n172 = Not(x=w492) -> (.not. x?=w493:bool)
              n173 = Divide(x=w490, y=i16 1000) -> (x/y=→"Battery":dbl)
              n174 = Wait Until Next ms Multiple(millisecond multiple=u32 100 ("milliseconds to wait")) -> ()  [unwired: 1 out]
              "How? 2" <- w492
            }
            n175 = while {
              shift-right: [w487] -> _
              shift-left: _ -> [w486]
              stop <- w485 stop-if-true
              # "ForebrainAct"
              n176 = local read "E-Stop"() -> (w483:bool)
              n177 = local read "ManualModeStop"() -> (w485:bool)
              n178 = Select(t=0.0, s=w483, f="Manual Vel") -> (s? t:f=w480:dbl)
              n179 = To Word Integer(number=w480) -> (16bit integer=w478:i16)
              "Speed" <- w478
              n180 = local read "Send String"() -> (→"Send String to NXT":string)
              n181 = To Word Integer(number="Behavior Command") -> (16bit integer=w475:i16)
              n182 = local write "Upper Midbrain Active"("Upper Midbrain Active") -> ()
              n183 = local write "Mode"(w475) -> ()
              n184 = local write "Desired \nVelocity"(w478) -> ()
              n185 = local write "Local\nHeading"("Manual Heading") -> ()
              n186 = Not(x=w486) -> (.not. x?=w487:bool)
              n187 = Wait Until Next ms Multiple(millisecond multiple=u32 50 ("milliseconds to wait")) -> ()  [unwired: 1 out]
              "ActManual" <- w486
            }
            n188 = local read "ManualModeStop"() -> (w436:bool)
            n189 = case shown="True" w436 {
              tunnel: [TRUE ("s") w497] -> w438
              tunnel: [T1."ManualMode" ("Tab") w498] -> w437
              frame False {
              }
              frame True {
                # "Debounce tab for clean transition"
                n190 = flat-sequence {
                  tunnel: [w504] -> w498
                  tunnel: [TRUE ("s")] -> w497
                  frame #0 {
                    n191 = Wait (ms)(milliseconds to wait=u32 100) -> ()  [unwired: 1 out]
                  }
                  frame #1 {
                    w504 = T1."Startup&Shutdown" ("Tab")
                    # "Turn off\nVelocity\non \nExit"
                    n192 = local write "ManualModeStop"(FALSE ("ManualModeStop")) -> ()
                    n193 = local write "Desired \nVelocity"(i16 0 ("Desired \nVelocity")) -> ()
                    n194 = local write "Local\nHeading"(i16 0 ("Local\nHeading")) -> ()
                    n195 = local write "Mode"(i16 0 ("Mode")) -> ()
                    n196 = local write "Tab"(w504) -> ()
                  }
                }
              }
            }
          }
          frame "AutoMode" {
            n197 = flat-sequence {
              tunnel: w512 -> [_]
              tunnel: [w515] -> w510
              tunnel: w509 -> [w515]
              tunnel: w508 -> [w514]
              tunnel: [w514] -> w507
              tunnel: w506 -> [_]
              tunnel: w510 -> [w522]
              tunnel: w507 -> [w520]
              tunnel: [w599] -> w513
              tunnel: [FALSE ("s")] -> w511
              frame #0 {
                # "Run Robot\nbased on\nmission\ndefinition\nfile"
                n198 = local write "AutoMissionMap"(w514) -> ()
                n199 = while {
                  shift-right: [w518] -> _
                  shift-left: _ -> [w517]
                  stop <- "RunAutoMode" continue-if-true
                  # "Wait for Run\nbutton press\nbefore\nturning on\nAutoMode\nCode"
                  n200 = Not(x=w517) -> (.not. x?=w518:bool)
                  n201 = Wait Until Next ms Multiple(millisecond multiple=u32 100 ("milliseconds to wait")) -> ()  [unwired: 1 out]
                  "Ready" <- w517
                }
              }
              frame #1 {
                n202 = while {
                  shift-right: [w568] -> _
                  shift-left: _ -> [w559]
                  tunnel: w522 -> [w563]
                  shift-right: [w561] -> _
                  shift-left: _ -> [w562]
                  tunnel: w520 -> [w554]
                  stop <- w558 stop-if-true
                  # "WhereAmI?"
                  n203 = local read "WhereAmI?FromBase"() -> (w553:T6)
                  n204 = Get Date/Time In Seconds "GetMiissionCurrentTime"() -> (seconds since 1Jan1904=w564:timestamp)
                  n205 = call "WhereForebrainPerception.vi"("Where? Midbrain"=w553) -> ("(xr,yr)"=w561:cluster{"X":dbl, "Y":dbl}, "Direction"=w547:dbl)  [unwired: 3 in, 2 out]
                  "Robot Position" <- w561
                  n206 = local read "RunAutoMode"() -> (w558:bool)
                  n207 = Greater Or Equal?(x=w547, y=181.0) -> (x >= y?=w551:bool)
                  n208 = To Double Precision Float(number=w564) -> (double precision float=w565:dbl)
                  n209 = Subtract(x=w565, y=w563) -> (x-y=w566:dbl)
                  n210 = Not(x=w559) -> (.not. x?=w568:bool)
                  n211 = call "DrawRobot.vi"("(xr,yr) old"=w562, "(xr,yr) new"=w561, "2D Picture"=w554) -> ("new picture"=→"AutoMissionMap":picture)
                  n212 = local read "SteerAngle"() -> (w556:dbl)
                  n213 = Divide(x=w566, y=60.0) -> (x/y=w560:dbl)
                  "MissionTimeAuto" <- w560
                  n214 = Subtract(x=w547, y=360.0) -> (x-y=w549:dbl)
                  n215 = Select(t=w549, s=w551, f=w547) -> (s? t:f=w548:dbl)
                  n216 = shared-variable "My Computer\\RobotBrainExLibrary.lvlib\\MissionTime"(w560) -> ()  [unwired: 1 in, 1 out]
                  n217 = Bundle("Direction"=w548, "SteerAngle"=w556) -> (→"A Heading":cluster{"Direction":dbl, "SteerAngle":dbl})  [unwired: 1 in]
                  n218 = Wait Until Next ms Multiple(millisecond multiple=u32 50 ("milliseconds to wait")) -> ()  [unwired: 1 out]
                  "Where?" <- w559
                }
                n219 = while {
                  shift-right: [w589] -> _
                  shift-left: _ -> [w588]
                  shift-right: [w571] -> _
                  shift-left: 0.0 ("SteerAngle") -> [w584]
                  stop <- w591 stop-if-true
                  # "needs to put out heading in local coordinates"
                  # "Think"
                  n220 = Not(x=w588) -> (.not. x?=w589:bool)
                  n221 = Or(x="Pause", y="E-Stop") -> (x .or. y?=w575:bool)
                  n222 = local read "WhereAmI?FromBase"() -> (w587:T6)
                  n223 = local read "WhatAroundMeMap?"() -> (w586:cluster{"T":dbl, "Range":dbl, "Bearing":dbl}[])
                  n224 = local read "MDF"() -> (w577:T4)
                  n225 = call "GotoWaypoint.vi"("InhibitIn"=w575, "CurrentSteerAngle"=w584, "WhatAroundMe? Clean"=w586, "WhereAmI? Clean"=w587, "MDF In"=w577) -> ("BehCom"=→"Current Behavior":T7, "MDF Out"=w579:T4, "ActCommand"=→"WayPointAct":dbl[], "Vel"=w572:dbl, "SteerAngle"=w571:dbl)  [unwired: 1 in, 1 out]
                  "SteerAngle" <- w571
                  "A Speed" <- w572
                  n226 = To Long Integer(number=w572) -> (32bit integer=w573:i32)
                  n227 = To Long Integer(number=w571) -> (32bit integer=w570:i32)
                  n228 = local write "MDF"(w579) -> ()
                  n229 = local write "Desired \nVelocity"(w573) -> ()
                  n230 = local read "RunAutoMode"() -> (w591:bool)
                  n231 = local write "Local\nHeading"(w570) -> ()
                  n232 = local read "MDF_Original"() -> (w582:T4)
                  n233 = local read "MDF"() -> (w581:T4)
                  n234 = Select(t=w582, s="Rerun MDF", f=w581) -> (s? t:f=w578:T4)
                  n235 = local write "MDF"(w578) -> ()
                  n236 = Wait Until Next ms Multiple(millisecond multiple=u32 50 ("milliseconds to wait")) -> ()  [unwired: 1 out]
                  "Neo-C" <- w588
                }
                n237 = while {
                  shift-right: [w540] -> _
                  shift-left: _ -> [w542]
                  stop <- w539 stop-if-true
                  # "WhatIsAroundMe?"
                  n238 = local read "WhatAroundMeMap?"() -> (w536:cluster{"T":dbl, "Range":dbl, "Bearing":dbl}[])
                  n239 = call "ProcessLidarData.vi"("WhatAroundMe?MM"=w536) -> ("Collision"=w537:bool, "data array [mag, phase (deg)]"=w541:cluster{"magnitude":dbl, "phase":dbl}[])
                  "CollisionLight 2" <- w537
                  n240 = local read "RunAutoMode"() -> (w539:bool)
                  n241 = call "SimLIDARPlot.vi"("data array [mag, phase (deg)]"=w541) -> ("SONAR"=→"AutoModeLIDAR":picture)  [unwired: 1 in]
                  n242 = Not(x=w542) -> (.not. x?=w540:bool)
                  "What?" <- w540
                  n243 = case shown="True" w537 {
                    frame False {
                      # "No \nBeep"
                    }
                    frame True {
                      n244 = call <vilib>:"Beep.vi"("use system alert? (T)"=TRUE, "duration (msec)"=u32 1000, "frequency (Hz)"=u32 900) -> ()  [unwired: 9 in]
                    }
                  }
                  n245 = Wait Until Next ms Multiple(millisecond multiple=u32 50 ("milliseconds to wait")) -> ()  [unwired: 1 out]
                }
                n246 = while {
                  shift-right: [w534] -> _
                  shift-left: _ -> [w533]
                  stop <- w532 stop-if-true
                  # "HowAmI?"
                  n247 = local read "Battery\nVolts"() -> (w530:i16)
                  n248 = local read "RunAutoMode"() -> (w532:bool)
                  n249 = Not(x=w533) -> (.not. x?=w534:bool)
                  n250 = Divide(x=w530, y=i16 1000) -> (x/y=→"AutoBattery":dbl)
                  n251 = Wait Until Next ms Multiple(millisecond multiple=u32 80 ("milliseconds to wait")) -> ()  [unwired: 1 out]
                  "How?" <- w533
                }
                n252 = while {
                  shift-right: [w527] -> _
                  shift-left: _ -> [w526]
                  stop <- w525 stop-if-true
                  # "calculate desired heading.vi"
                  # "see calc desired\nheading"
                  # "convert to \noutputtin\nDesired v and\nlocal heading"
                  # "chnage arbiter to be -180 to 180"
                  # "Note:\nadd other beh to\narbiter"
                  # "ForebrainAct"
                  n253 = local read "WayPointAct"() -> (w524:dbl[])
                  n254 = local read "RunAutoMode"() -> (w525:bool)
                  n255 = Not(x=w526) -> (.not. x?=w527:bool)
                  n256 = call "ForebrainArbiter.vi"("WaypointInput"=w524) -> ("ForebrainActCom"=w523:dbl[])  [unwired: 14 in]
                  n257 = shared-variable "My Computer\\RobotBrainExLibrary.lvlib\\ActCommand"(w523) -> ()  [unwired: 1 in, 1 out]
                  n258 = Wait Until Next ms Multiple(millisecond multiple=u32 50 ("milliseconds to wait")) -> ()  [unwired: 1 out]
                  "Act" <- w526
                }
              }
              frame #2 {
                w599 = T1."Startup&Shutdown" ("Tab")
                # "Set robot Vel to 0"
                # "Reset latched run\nswitch"
                # "Force control to\nShutdown Case"
                n259 = shared-variable "My Computer\\RobotBrainExLibrary.lvlib\\ForebrainCom"(T8 {"VelCom"=0.0, "BehCom"=enum."OpenFieldTransit"} ("ForebrainCom")) -> ()  [unwired: 1 in, 1 out]
                n260 = local write "RunAutoMode"(TRUE ("RunAutoMode")) -> ()
                n261 = Initialize Array(0.0 ("element"), 90 ("dimension size")) -> (w595:dbl[])
                n262 = shared-variable "My Computer\\RobotBrainExLibrary.lvlib\\ActCommand"(w595) -> ()  [unwired: 1 in, 1 out]
                n263 = shared-variable "My Computer\\RobotBrainExLibrary.lvlib\\Xstart"(200.0 ("Xstart")) -> ()  [unwired: 1 in, 1 out]
                n264 = shared-variable "My Computer\\RobotBrainExLibrary.lvlib\\Ystart"(400.0 ("Ystart")) -> ()  [unwired: 1 in, 1 out]
                n265 = local write "Tab"(w599) -> ()
              }
            }
          }
          frame "Documentation" {
            # "Add:\n1) Blinking lights in each loop to show that they are running"
            # "This mode is just a static data flow picture of the ForeBrain"
            n266 = Wait (ms)(milliseconds to wait=u32 500) -> ()  [unwired: 1 out]
          }
          frame "DebugTHINK" {
            w609 = T1."Startup&Shutdown" ("Tab")
            # "Add:\n1) a button for each midbrain behavior to help in debugging\n2) graph of \"neural\" arbiter brain waves for each actuator\n3) a button for each forebrain behavior"
            # "Put code here in place of delay"
            # "Sends Tab Control\nback to Startup\ncase"
            n267 = Wait (ms)(milliseconds to wait=u32 5000) -> ()  [unwired: 1 out]
            n268 = local write "Tab"(w609) -> ()
          }
        }
        n269 = Not(x=w192) -> (.not. x?=w175:bool)
        "Robot Live" <- w175
      }
      n270 = while {
        tunnel: w56 -> [w159]
        tunnel: w55 -> [w158]
        tunnel: [w157] -> w53
        tunnel: [w156] -> w54
        shift-right: [w150] -> _
        shift-left: _ -> [w149]
        stop <- w160 continue-if-true
        w162 = 250  # timeout
        # "Finds and displays tugs position"
        # "runs continuously till program stops"
        # "Comminications with Base Station"
        # "receive string"
        # "If time out, post timeout and\nremove the timeout error"
        # "Read data from the port."
        n271 = Wait Until Next ms Multiple(millisecond multiple=u32 1) -> ()  [unwired: 1 out]
        n272 = UDP Read(connection ID=w159, timeout ms (25000)=w162, 8:w158) -> (data out=w151:string, error out=w163:errorcluster, 3:w156:refnum<k16>)  [unwired: 1 in, 2 out]
        n273 = local write "Base Station data rec'd"(w151) -> ()
        n274 = Unbundle By Name(w163) -> ("code"=w166:i32)
        n275 = Equal?(x=w166, y=56) -> (x = y?=w164:bool)
        "BS Time Out?" <- w164
        n276 = case shown="True" w164 {
          tunnel: [w173 errorcluster {"status"=FALSE, "code"=0, "source"=""} ("error out")] -> w157
          tunnel: w163 -> [w173 _]
          frame False {
          }
          frame True {
          }
        }
        n277 = call "PC parse the data.vi"("Nav String"=w151, "Tug"="Tug letter") -> ("Buoy locations"=w155:cluster{"regular expression":string, i32, i32}[], "Tug Location"=w153:T13, "Valid?"=w154:bool)  [unwired: 1 out]
        "Valid ?" <- w154
        n278 = local write "Buoy locations"(w155) -> ()
        n279 = case shown="True" w154 {
          tunnel: w153 -> [_ w172]
          frame False {
            # "No \nchange"
          }
          frame True {
            # "New values from BaseStation"
            n280 = shared-variable "My Computer\\RobotBrainExLibrary.lvlib\\MissionTime"() -> (w171:dbl)  [unwired: 1 in, 1 out]
            n281 = Unbundle(w172) -> (w170:i32, w169:i32, w168:i32)  [unwired: 1 out]
            n282 = local write "Tug X"(w170) -> ()
            n283 = local write "Tug Y"(w169) -> ()
            n284 = local write "Tug H"(w168) -> ()
            n285 = Bundle(w171, w170, w169, w168) -> (w167:cluster{dbl, i32, i32, i32})  [unwired: 1 in]
            n286 = local write "WhereAmI?FromBase"(w167) -> ()
          }
        }
        n287 = local read "RunRobot"() -> (w160:bool)
        n288 = Not(x=w149) -> (.not. x?=w150:bool)
        "udp rate" <- w149
      }
      n289 = while {
        tunnel: w57 -> [_]
        stop <- w99 continue-if-true
        n290 = local read "Upper Midbrain Active"() -> (w98:bool)
        n291 = case shown="True" w98 {
          frame False {
            # "loop timimng \ncontrolled externally"
            # "Send commands to NXT"
            n292 = local read "Desired \nVelocity"() -> (w110:i16)
            n293 = local read "Local\nHeading"() -> (w109:i16)
            n294 = local read "Mode"() -> (w108:i16)
            n295 = case shown="2" w108 {
              tunnel: w110 -> [w113 w124 w131]
              tunnel: w109 -> [w112 w123 w132]
              tunnel: [w114 w119 w127] -> w102
              tunnel: i16 7 ("element") -> [w111 w120 w128]
              frame 0, Default {
                w115 = i16 0 ("element")
                n296 = Build Array(u8 91 ("element"), w111, w112, w113, i16 1 ("element"), w115, w115, w115, w115, w115, u8 93 ("element")) -> (w114:i16[])
              }
              frame 1 {
                w121 = i16 0 ("element")
                n297 = Build Array(u8 91 ("element"), w120, w123, w124, w121, i16 1 ("element"), w121, w121, w121, w121, u8 93 ("element")) -> (w119:i16[])
              }
              frame 2 {
                w129 = i16 0 ("element")
                n298 = Build Array(u8 91 ("element"), w128, w132, w131, w129, w129, i16 1 ("element"), w129, w129, w129, u8 93 ("element")) -> (w127:i16[])
              }
            }
            n299 = Select(t=u8[] [91, 7, 7, 7, 1, 0, 0, 0, 0, 0, 92], s="Soft E-Stop", f=w102) -> (s? t:f=w103:i16[])
            n300 = Add(x=w103, y=u8[] [0, 65, 65, 65, 65, 65, 65, 65, 65, 65, 0]) -> (x+y=w104:i16[])
            n301 = Byte Array To String(unsigned byte array=w104) -> (string=w101:string)
            n302 = local write "Send String"(w101) -> ()
          }
          frame True {
            n303 = local read "ManualModeStop"() -> (w136:bool)
            n304 = call "UpperMidbrain.vi"("SOFT E-STOP"=w136, "IR Servo"=u8 7) -> ("string"=w137:string)  [unwired: 9 in]
            n305 = local write "Send String"(w137) -> ()
          }
        }
        n306 = local read "RunRobot"() -> (w99:bool)
      }
      n307 = while {
        tunnel: w57 -> [_]
        stop <- w76 continue-if-true
        # "Receive information from NXT"
        n308 = local read "String Received"() -> (w81:string)
        n309 = Wait Until Next ms Multiple(millisecond multiple=u32 100) -> ()  [unwired: 1 out]
        n310 = String Subset(string=w81, offset (0)=1, length (rest)=1 ("length (rest)")) -> (substring=w80:string)
        n311 = case shown="\"N\"" w80 {
          tunnel: w81 -> [_ w83]
          frame Default {
          }
          frame "N" {
            # "0-15"
            # "Parse command \"N\""
            n312 = String Subset(string=w83, offset (0)=2, length (rest)=4 ("length (rest)")) -> (substring=w94:string)
            n313 = String Subset(string=w83, offset (0)=6, length (rest)=3 ("length (rest)")) -> (substring=w90:string)
            n314 = String Subset(string=w83, offset (0)=9, length (rest)=2 ("length (rest)")) -> (substring=w86:string)
            n315 = Decimal String To Number(string=w94) -> (number=w97:i32)  [unwired: 2 in, 1 out]
            n316 = Decimal String To Number(string=w90) -> (number=w89:i32)  [unwired: 2 in, 1 out]
            n317 = Decimal String To Number(string=w86) -> (number=w87:i32)  [unwired: 2 in, 1 out]
            n318 = To Word Integer(number=w97) -> (16bit integer=w93:i16)
            n319 = To Word Integer(number=w89) -> (16bit integer=w88:i16)
            n320 = To Long Integer(number=w87) -> (32bit integer=w82:i32)
            n321 = local write "LidarDist"(w88) -> ()
            n322 = local write "Battery\nVolts"(w93) -> ()
            n323 = local write "IR Index"(w82) -> ()
          }
        }
        n324 = local read "RunRobot"() -> (w76:bool)
      }
      n325 = while {
        stop <- w75 continue-if-true
        # "Run Simulated MapDAR"
        n326 = local read "Tug X"() -> (w73:i32)
        n327 = local read "Tug Y"() -> (w72:i32)
        n328 = local read "Tug H"() -> (w71:i32)
        n329 = Bundle "Bundle"("Tug X"=w73, "Tug Y"=w72, "Tug H"=w71) -> (w74:cluster{"Tug X":i32, "Tug Y":i32, "Tug H":i32})  [unwired: 1 in]
        n330 = call "HindbrainLIDAR_Sim.vi"("SubPosition"=w74) -> ("WhatAroundMe?"=→"WhatAroundMeMap?":cluster{"T":dbl, "Range":dbl, "Bearing":dbl}[])  [unwired: 10 in]
        n331 = local read "RunRobot"() -> (w75:bool)
      }
    }
    frame #2 {
      # "Close XBee Radio"
      # "Close UDP port"
      # "Realease LIDAR\nMemory"
      # "Reset Run \nSwitch"
      # "Shutdown Robot"
      n332 = call "Pixel_LIDAR_Close.vi"("error in (no error) 2"=w615, "Image"=w616) -> ()  [unwired: 1 in]
      n333 = local write "RunRobot"(TRUE ("RunRobot")) -> ()
      n334 = call "XB PC Close.vi"("error in (no error)"=w613, "VISA resource name"=w614) -> ()
      n335 = UDP Close(connection ID=w612, 8:w611) -> ()  [unwired: 2 out]
      "error out" <- w613
    }
  }
